vi "checkifDisconnectsubVI.vi"(10 "port_number in":string, 11 "function return 3":i32) -> ()   [LabVIEW 2012]
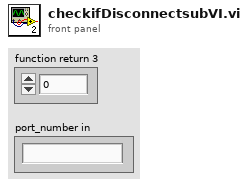
[diagram p1: front panel]
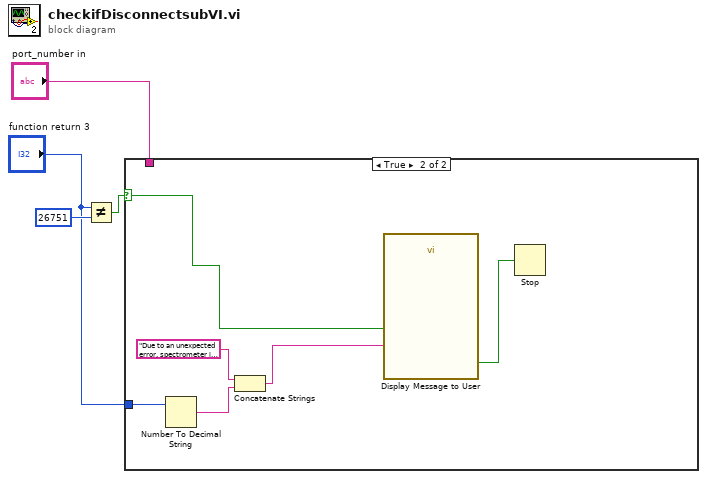
[diagram p0: block diagram]
diagram:
  n1 = Not Equal?(x="function return 3", y=26751) -> (x != y?=w1:bool)
  n2 = case shown="True" w1 {
    selector: w1 -> [_ w5]
    tunnel: "port_number in" -> [_ _]
    tunnel: "function return 3" -> [_ w9]
    frame False {
    }
    frame True {
      n3 = Number To Decimal String(number=w9) -> (decimal integer string=w8:string)  [unwired: 1 in]
      n4 = Concatenate Strings("Due to an unexpected error, spectrometer is disconnected and the program has been stopped. Please rerun the program and reconnect. Probably, data is incomplete.\n\nFor this data format;\n\nExpected number of bytes: 26751\n\nRead number of bytes: ", w8) -> (w7:string)
      n5 = call "Display Message to User"("Enable"=w5, "Message"=w7) -> ("OK"=w10:bool)  [unwired: 8 in, 1 out]
      n6 = Stop(stop? (T)=w10) -> ()
    }
  }
